vi "SVPO Average FFT Spectrum (Complex).vi"   [LabVIEW 2017]
doc: "Converts a frequency power spectrum to an order power spectrum. Use this VI to convert power spectrum results from constant-speed applications."
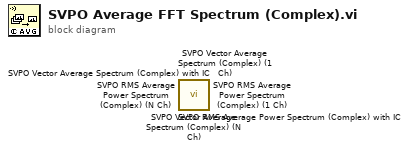
[diagram p0: block diagram]
diagram:
  n1 = call <vilib>:"SVPO Vector Average Spectrum (Complex) (N Ch).vi"() -> ()  [unwired: 18 in, 2 out]
  n2 = call <vilib>:"SVPO Vector Average Spectrum (Complex) (1 Ch).vi"() -> ()  [unwired: 18 in, 2 out]
  n3 = call <vilib>:"SVPO RMS Average Power Spectrum (Complex) (N Ch).vi"() -> ()  [unwired: 17 in, 3 out]
  n4 = call <vilib>:"SVPO RMS Average Power Spectrum (Complex) (1 Ch).vi"() -> ()  [unwired: 17 in, 3 out]
  n5 = call <vilib>:"SVPO Vector Average Spectrum (Complex) with IC.vi"() -> ()  [unwired: 18 in, 2 out]
  n6 = call <vilib>:"SVPO RMS Average Power Spectrum (Complex) with IC.vi"() -> ()  [unwired: 17 in, 3 out]
